vi "createUserEvents.vi"(8 "error in (no error)":errorcluster) -> (0 "error out":errorcluster, 3 "userEvents":T1)   [LabVIEW 2017, in "User Event - Stop.lvlib"]
doc: "Create a boolean user event that will be used to stop the event loop from the message handling loop."
uses:
  User Event - Stop.lvlib
  userEvents.ctl
  Controls/objectRefsMain.ctl
  sendRefs.ctl
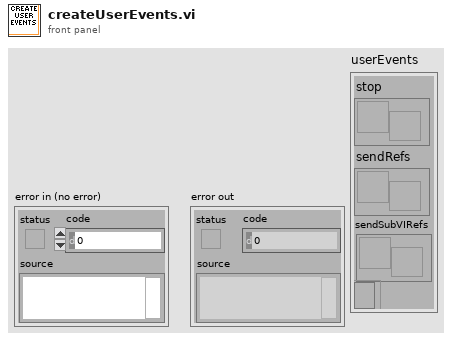
[diagram p1: front panel]
types:
  T1 = typedef "User Event - Stop.lvlib/userEvents.ctl" = cluster{"stop":refnum<user-event>, "sendRefs":refnum<user-event>, "sendSubVIRefs":refnum<user-event>, "eventRegRef":refnum<event-registration>}
  T2 = typedef "User Event - Stop.lvlib/sendRefs.ctl" = cluster{"objectRefsMain":T3}
  T3 = typedef "objectRefsMain.ctl" = cluster{"experiorLogoRef":refnum<vi>, "menuSplitter1Ref":refnum<vi>, "moduleSplitter1Ref":refnum<vi>, "moduleSplitter2Ref":refnum<vi>, "statusMessageSplitterRef":refnum<vi>, "logoSplitter1Ref":refnum<vi>, "logoSplitter2Ref":refnum<vi>, "logoPaneRef":refnum<vi>, "titlePaneRef":refnum<vi>, "menuPane1Ref":refnum<vi>, "modulePane1Ref":refnum<vi>, "modulePane2Ref":refnum<vi>, "modulePane3Ref":refnum<vi>, "statusMessagePaneRef":refnum<vi>, "abortRef":refnum<vi>, "menuSliderRef":refnum<vi>, "moduleSliderRef":refnum<vi>, "statusMessageRef":refnum<vi>, "SubVISubpanelRef":refnum<vi>, "moduleSplitter3Ref":refnum<vi>, "modulePane4Ref":refnum<vi>, "deviceIdRef":refnum<vi>, "SaveFileRef":refnum<vi>, "SampleIDRef":refnum<vi>, "ChannelRef":refnum<vi>, "UseSwitchRef":refnum<vi>, "MeasButtonRef":refnum<vi>, "RefButtonRef":refnum<vi>, "SaveButtonRef":refnum<vi>, "EnlableIlRef":refnum<vi>, "EnlableRlRef":refnum<vi>, "WavelengthRef":refnum<vi>, "ChannelClusterRef":refnum<vi>, "RunTimeRef":refnum<vi>, "RereferenceRef":refnum<vi>, "RemeasureRef":refnum<vi>, "EngModeRef":refnum<vi>, "StandardSelectRef":refnum<vi>, "MethodSelectRef":refnum<vi>, "StandardRef":refnum<vi>, "SavePathRef":refnum<vi>}
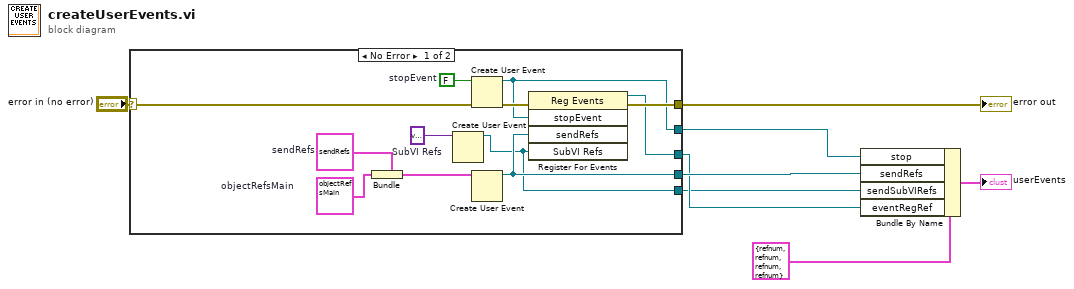
[diagram p0: block diagram]
diagram:
  n1 = case shown="No Error" "error in (no error)" {
    selector: "error in (no error)" -> [w19 w21]
    tunnel: [w16 _] -> w6
    tunnel: [w17 w21] -> w8
    tunnel: [w15 _] -> w2
    tunnel: [w14 _] -> w5
    tunnel: [w9 _] -> w1
    frame No Error {
      w10 = variant  # SubVI Refs
      w11 = T2 {"objectRefsMain"={"experiorLogoRef"=refnum, "menuSplitter1Ref"=refnum, "moduleSplitter1Ref"=refnum, "moduleSplitter2Ref"=refnum, "statusMessageSplitterRef"=refnum, "logoSplitter1Ref"=refnum, "logoSplitter2Ref"=refnum, "logoPaneRef"=refnum, "titlePaneRef"=refnum, "menuPane1Ref"=refnum, "modulePane1Ref"=refnum, "modulePane2Ref"=refnum, "modulePane3Ref"=refnum, "statusMessagePaneRef"=refnum, "abortRef"=refnum, "menuSliderRef"=refnum, "moduleSliderRef"=refnum, "statusMessageRef"=refnum, "SubVISubpanelRef"=refnum, "moduleSplitter3Ref"=refnum, "modulePane4Ref"=refnum, "deviceIdRef"=refnum, "SaveFileRef"=refnum, "SampleIDRef"=refnum, "ChannelRef"=refnum, "UseSwitchRef"=refnum, "MeasButtonRef"=refnum, "RefButtonRef"=refnum, "SaveButtonRef"=refnum, "EnlableIlRef"=refnum, "EnlableRlRef"=refnum, "WavelengthRef"=refnum, "ChannelClusterRef"=refnum, "RunTimeRef"=refnum, "RereferenceRef"=refnum, "RemeasureRef"=refnum, "EngModeRef"=refnum, "StandardSelectRef"=refnum, "MethodSelectRef"=refnum, "StandardRef"=refnum, "SavePathRef"=refnum}}  # sendRefs
      w13 = T3 {"experiorLogoRef"=refnum, "menuSplitter1Ref"=refnum, "moduleSplitter1Ref"=refnum, "moduleSplitter2Ref"=refnum, "statusMessageSplitterRef"=refnum, "logoSplitter1Ref"=refnum, "logoSplitter2Ref"=refnum, "logoPaneRef"=refnum, "titlePaneRef"=refnum, "menuPane1Ref"=refnum, "modulePane1Ref"=refnum, "modulePane2Ref"=refnum, "modulePane3Ref"=refnum, "statusMessagePaneRef"=refnum, "abortRef"=refnum, "menuSliderRef"=refnum, "moduleSliderRef"=refnum, "statusMessageRef"=refnum, "SubVISubpanelRef"=refnum, "moduleSplitter3Ref"=refnum, "modulePane4Ref"=refnum, "deviceIdRef"=refnum, "SaveFileRef"=refnum, "SampleIDRef"=refnum, "ChannelRef"=refnum, "UseSwitchRef"=refnum, "MeasButtonRef"=refnum, "RefButtonRef"=refnum, "SaveButtonRef"=refnum, "EnlableIlRef"=refnum, "EnlableRlRef"=refnum, "WavelengthRef"=refnum, "ChannelClusterRef"=refnum, "RunTimeRef"=refnum, "RereferenceRef"=refnum, "RemeasureRef"=refnum, "EngModeRef"=refnum, "StandardSelectRef"=refnum, "MethodSelectRef"=refnum, "StandardRef"=refnum, "SavePathRef"=refnum}  # objectRefsMain
      w20 = FALSE  # stopEvent
      n2 = Bundle(cluster=w11, "objectRefsMain"=w13) -> (w12:T2)
      n3 = Create User Event(user event datatype=w10) -> (user event=w9:refnum<user-event>)  [unwired: 1 in, 1 out]
      n4 = Create User Event(user event datatype=w20, error in=w19) -> (user event=w16:refnum<user-event>, error out=w18:errorcluster)
      n5 = Create User Event(user event datatype=w12) -> (user event=w14:refnum<user-event>)  [unwired: 1 in, 1 out]
      n6 = register-events(error in=w18, w16, w14, w9) -> (reference out=w15:refnum<event-registration>, error out=w17:errorcluster)  [unwired: 1 in]
    }
    frame Error {
    }
  }
  "error out" <- w8
  n7 = Bundle By Name(cluster=T1 {"stop"=refnum, "sendRefs"=refnum, "sendSubVIRefs"=refnum, "eventRegRef"=refnum} ("userEvents"), "stop"=w6, "sendRefs"=w5, "sendSubVIRefs"=w1, "eventRegRef"=w2) -> (→"userEvents":T1)
